vi "Virbration SequenceFGV.vi"(1 "Action":T3(ring)=enum."Add", 5 "X":i32, 7 "VirbSeqData":T1, 9 "DataIn":string, 11 "error in":errorcluster) -> (4 "VirbSeqDataList":T2(array[cluster]), 6 "VirbSeqData":T1, 15 "error out":errorcluster)   [LabVIEW 2019]
uses:
  09bdc40f-24f8-42fa-be14-94a5734f4f81.vi
  3a88f7dc-0fdf-4cec-95e5-a4f3429e1c34.vi
  LLB/Commonly VI/Main Glb.vi
  <vilib>/JDP Science/JSONtext/Variant to JSON Text.vi
  <vilib>/JDP Science/JSONtext/JSON text to Variant.vi
  LLB/Commonly VI.lvlib
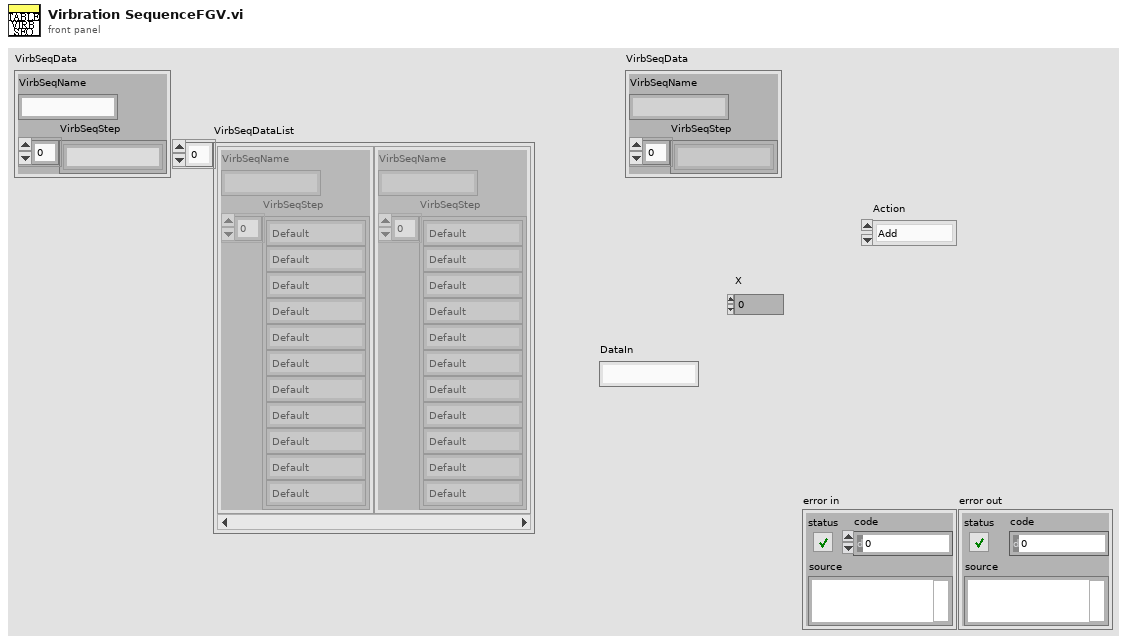
[diagram p1: front panel]
types:
  T1 = cluster{"VirbSeqName":string, "VirbSeqStep":string[]}
  T2 = cluster{"VirbSeqName":string, "VirbSeqStep":string[]}[]
  T3 = enum16{"Initial", "Write", "Read", "Save", "Load", "Add", "Delete"}
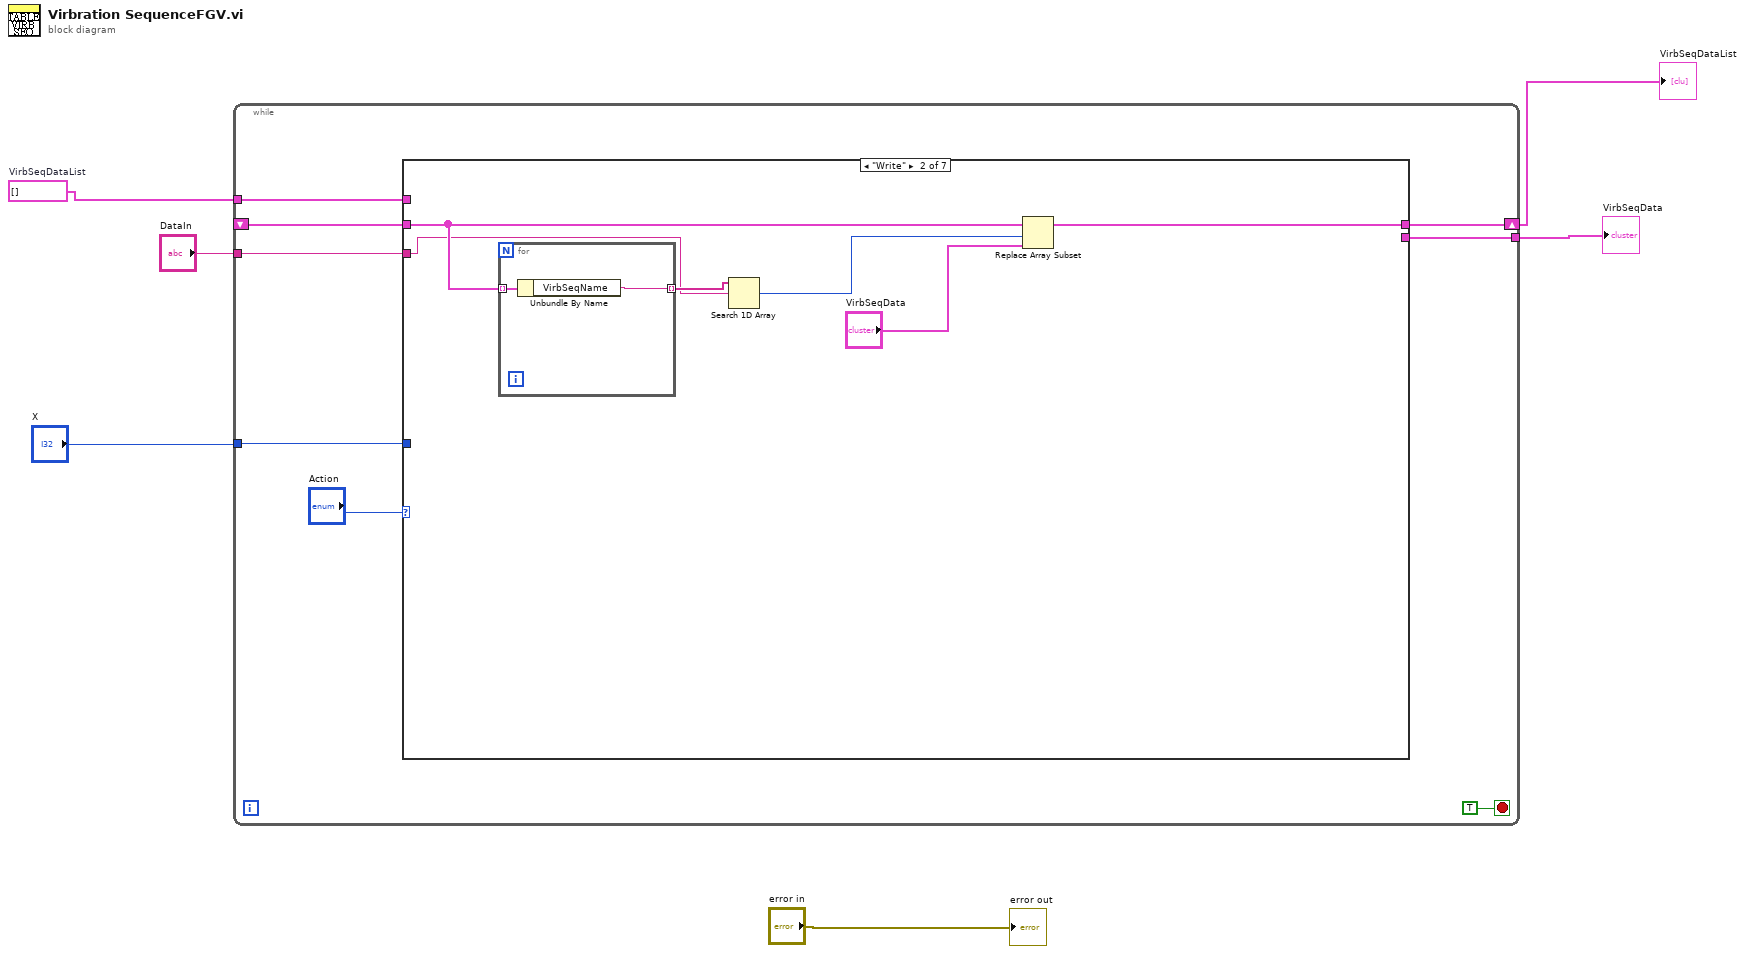
[diagram p0: block diagram]
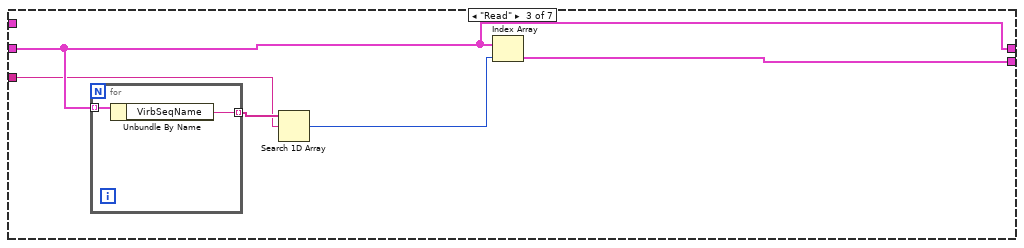
[diagram p3: hidden frame]
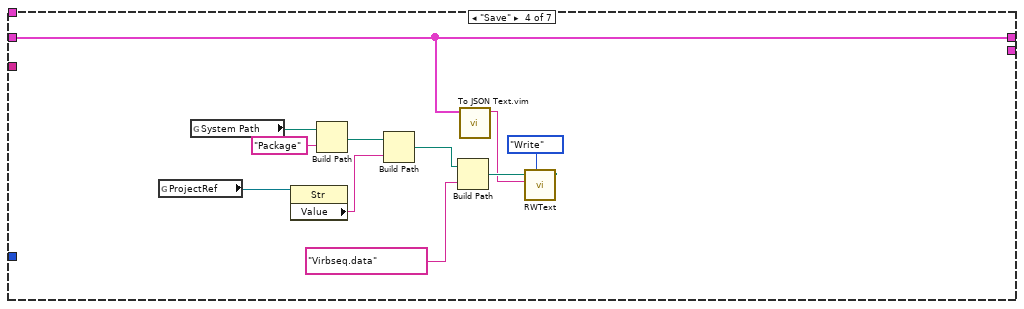
[diagram p4: hidden frame]
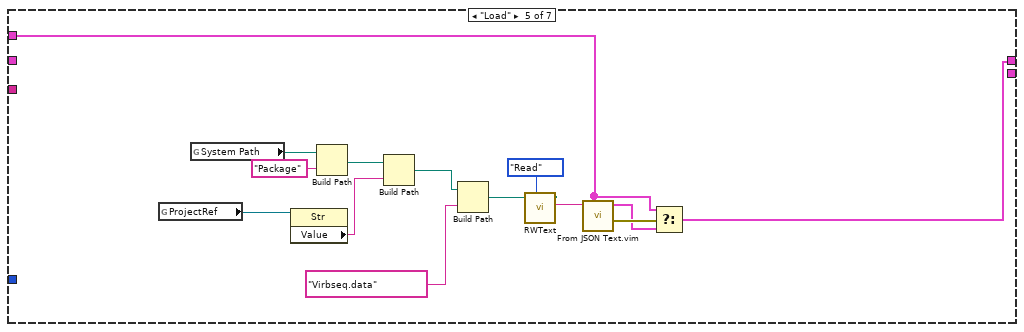
[diagram p5: hidden frame]
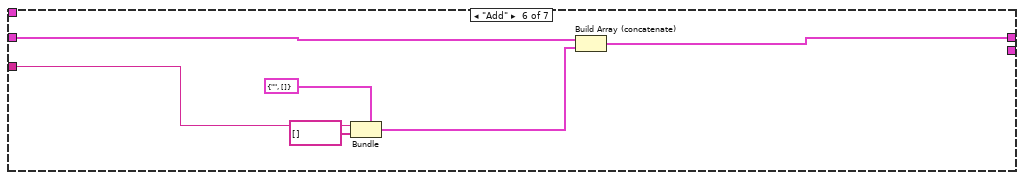
[diagram p6: hidden frame]
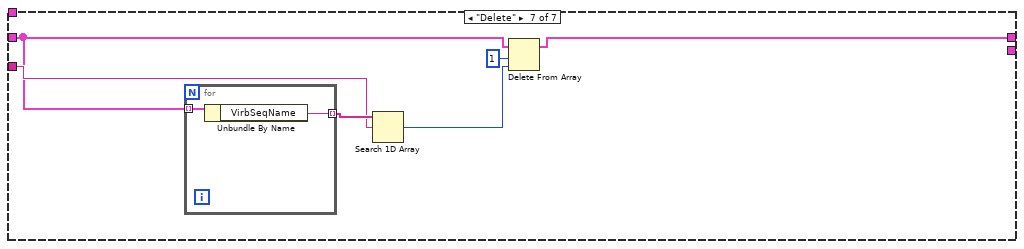
[diagram p7: hidden frame]
diagram:
  w3 = T2 []  # VirbSeqDataList
  n1 = while {
    shift-right: [w14] -> w2
    shift-left: _ -> [w13]
    tunnel: w3 -> [w12]
    tunnel: "X" -> [w10]
    tunnel: "DataIn" -> [w9]
    tunnel: [w7] -> w1
    stop <- TRUE stop-if-true
    n2 = case shown="\"Write\"" "Action" {
      tunnel: [w15 w21 w27 w32 w42 w60 w62] -> w14
      tunnel: w13 -> [_ w19 w27 w32 _ w61 w65]
      tunnel: w12 -> [w15 _ _ _ w44 _ _]
      tunnel: w10 -> [_ _ _ _ _ _ _]
      tunnel: w9 -> [_ w17 w25 _ _ w57 w66]
      tunnel: [_ _ w28 _ _ _ _] -> w7
      frame "Initial", Default {
      }
      frame "Write" {
        n3 = for {
          tunnel: w19 -> [w23] mode=indexing
          tunnel: [w22] -> w18 mode=indexing
          n4 = Unbundle By Name(w23) -> ("VirbSeqName"=w22:string)
        }
        n5 = Search 1D Array(1D array=w18, element=w17) -> (index of element=w16:i32)  [unwired: 1 in]
        n6 = Replace Array Subset(array=w19, new element="VirbSeqData", index=w16) -> (w21:T2)
      }
      frame "Read" {
        n7 = for {
          tunnel: w27 -> [w30] mode=indexing
          tunnel: [w29] -> w26 mode=indexing
          n8 = Unbundle By Name(w30) -> ("VirbSeqName"=w29:string)
        }
        n9 = Search 1D Array(1D array=w26, element=w25) -> (index of element=w24:i32)  [unwired: 1 in]
        n10 = Index Array(array=w27, index=w24) -> (element=w28:T1)
      }
      frame "Save" {
        n11 = global read "Main Glb.vi" "ProjectRef"() -> (w38:refnum<vi>)
        n12 = global read "Main Glb.vi" "System Path"() -> (w41:path)
        n13 = property class="Str"(reference=w38) -> ("Value"=w37:string)  [unwired: 1 in, 2 out]
        n14 = Build Path(base path=w41, name or relative path="Package") -> (appended path=w39:path)
        n15 = Build Path(base path=w39, name or relative path=w37) -> (appended path=w35:path)
        n16 = Build Path(base path=w35, name or relative path="Virbseq.data") -> (appended path=w33:path)
        n17 = call "To JSON Text.vim"("Anything"=w32) -> ("<JSON>"=w31:string)  [unwired: 9 in, 1 out]
        n18 = call "RWText.vi"("Action"=enum16{"Read", "Write"}."Write", "TextIn"=w31, "file path (use dialog)"=w33) -> ()  [unwired: 7 in, 2 out]
      }
      frame "Load" {
        n19 = global read "Main Glb.vi" "ProjectRef"() -> (w52:refnum<vi>)
        n20 = global read "Main Glb.vi" "System Path"() -> (w55:path)
        n21 = property class="Str"(reference=w52) -> ("Value"=w51:string)  [unwired: 1 in, 2 out]
        n22 = Build Path(base path=w55, name or relative path="Package") -> (appended path=w53:path)
        n23 = Build Path(base path=w53, name or relative path=w51) -> (appended path=w49:path)
        n24 = Build Path(base path=w49, name or relative path="Virbseq.data") -> (appended path=w47:path)
        n25 = call "RWText.vi"("Action"=enum16{"Read", "Write"}."Read", "file path (use dialog)"=w47) -> ("textOut"=w46:string)  [unwired: 8 in, 1 out]
        n26 = call "From JSON Text.vim"("Data Type and Default Value"=w44, "JSON"=w46) -> ("error out"=w45:errorcluster, "Data out"=w43:T2)  [unwired: 8 in]
        n27 = Select(t=w44, s=w45, f=w43) -> (s? t:f=w42:T2)
      }
      frame "Add" {
        n28 = Bundle(cluster=T1 {"VirbSeqName"="", "VirbSeqStep"=[]}, "VirbSeqName"=w57, "VirbSeqStep"=string[] []) -> (w58:T1)
        n29 = Build Array (concatenate)(w61, w58) -> (w60:T2)
      }
      frame "Delete" {
        n30 = for {
          tunnel: w65 -> [w69] mode=indexing
          tunnel: [w68] -> w67 mode=indexing
          n31 = Unbundle By Name(w69) -> ("VirbSeqName"=w68:string)
        }
        n32 = Search 1D Array(1D array=w67, element=w66) -> (index of element=w64:i32)  [unwired: 1 in]
        n33 = Delete From Array(array=w65, length=1, index=w64) -> (array with subset deleted=w62:T2)  [unwired: 1 out]
      }
    }
  }
  "VirbSeqDataList" <- w2
  "VirbSeqData" <- w1
  "error out" <- "error in"
